vi "Gather image parameters.vi"(8 "error in":errorcluster, 11 "Acq params":T1) -> (0 "error out":errorcluster, 3 "Acqusition string":string)   [LabVIEW 2018]
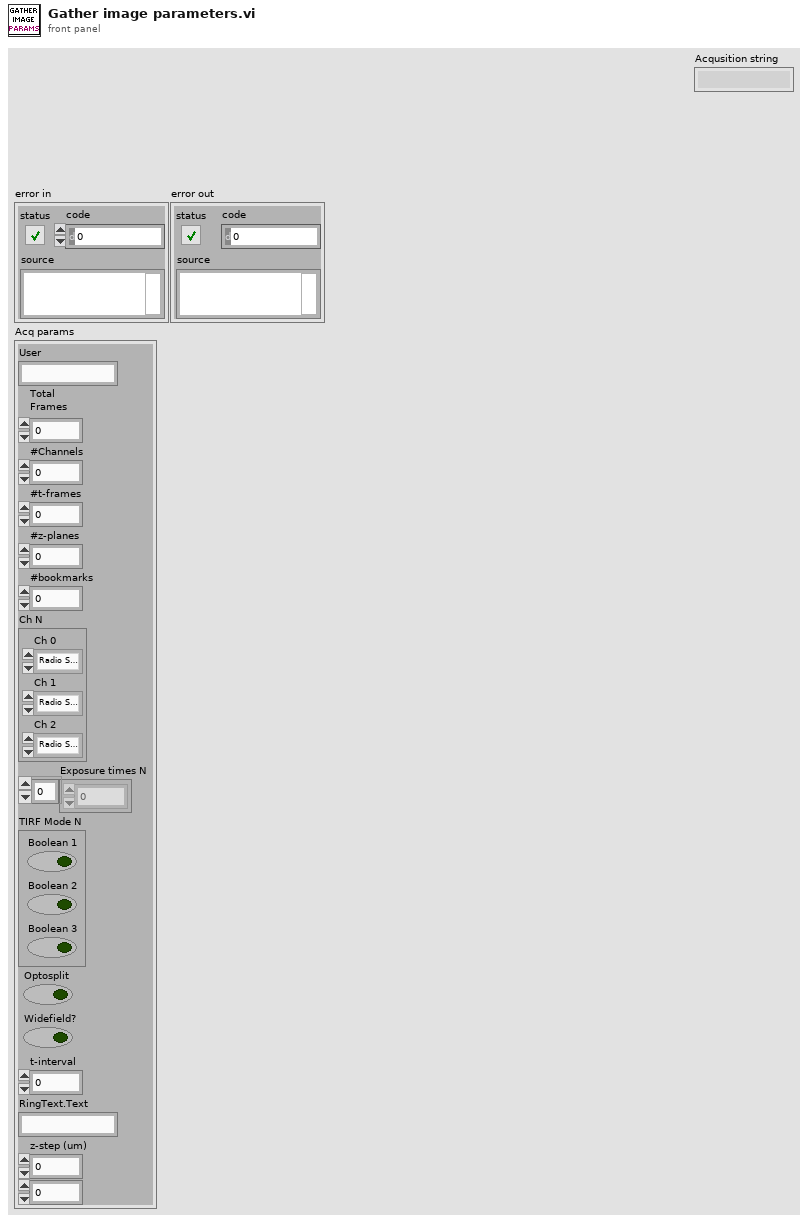
[diagram p1: front panel]
types:
  T1 = cluster{"User":string, "Total\nFrames":i16, "#Channels":i16, "#t-frames":i16, "#z-planes":i16, "#bookmarks":i16, "Ch N":cluster{"Ch 0":enum32{"Radio Selection 1", "Radio Selection 2", "Radio Selection 3"}, "Ch 1":enum32{"Radio Selection 1", "Radio Selection 2", "Radio Selection 3"}, "Ch 2":enum32{"Radio Selection 1", "Radio Selection 2", "Radio Selection 3"}}, "Exposure times N":dbl[], "TIRF Mode N":cluster{"Boolean 1":bool, "Boolean 2":bool, "Boolean 3":bool}, "Optosplit":bool, "Widefield?":bool, "t-interval":u32, "RingText.Text":string, "z-step (um)":dbl, i32}
  T2 = cluster{"Ch 0":enum32{"Radio Selection 1", "Radio Selection 2", "Radio Selection 3"}, "Ch 1":enum32{"Radio Selection 1", "Radio Selection 2", "Radio Selection 3"}, "Ch 2":enum32{"Radio Selection 1", "Radio Selection 2", "Radio Selection 3"}}
  T3 = cluster{"Boolean 1":bool, "Boolean 2":bool, "Boolean 3":bool}
  T4 = enum32{"Radio Selection 1", "Radio Selection 2", "Radio Selection 3"}
  T5 = enum32{"Radio Selection 1", "Radio Selection 2", "Radio Selection 3"}[]
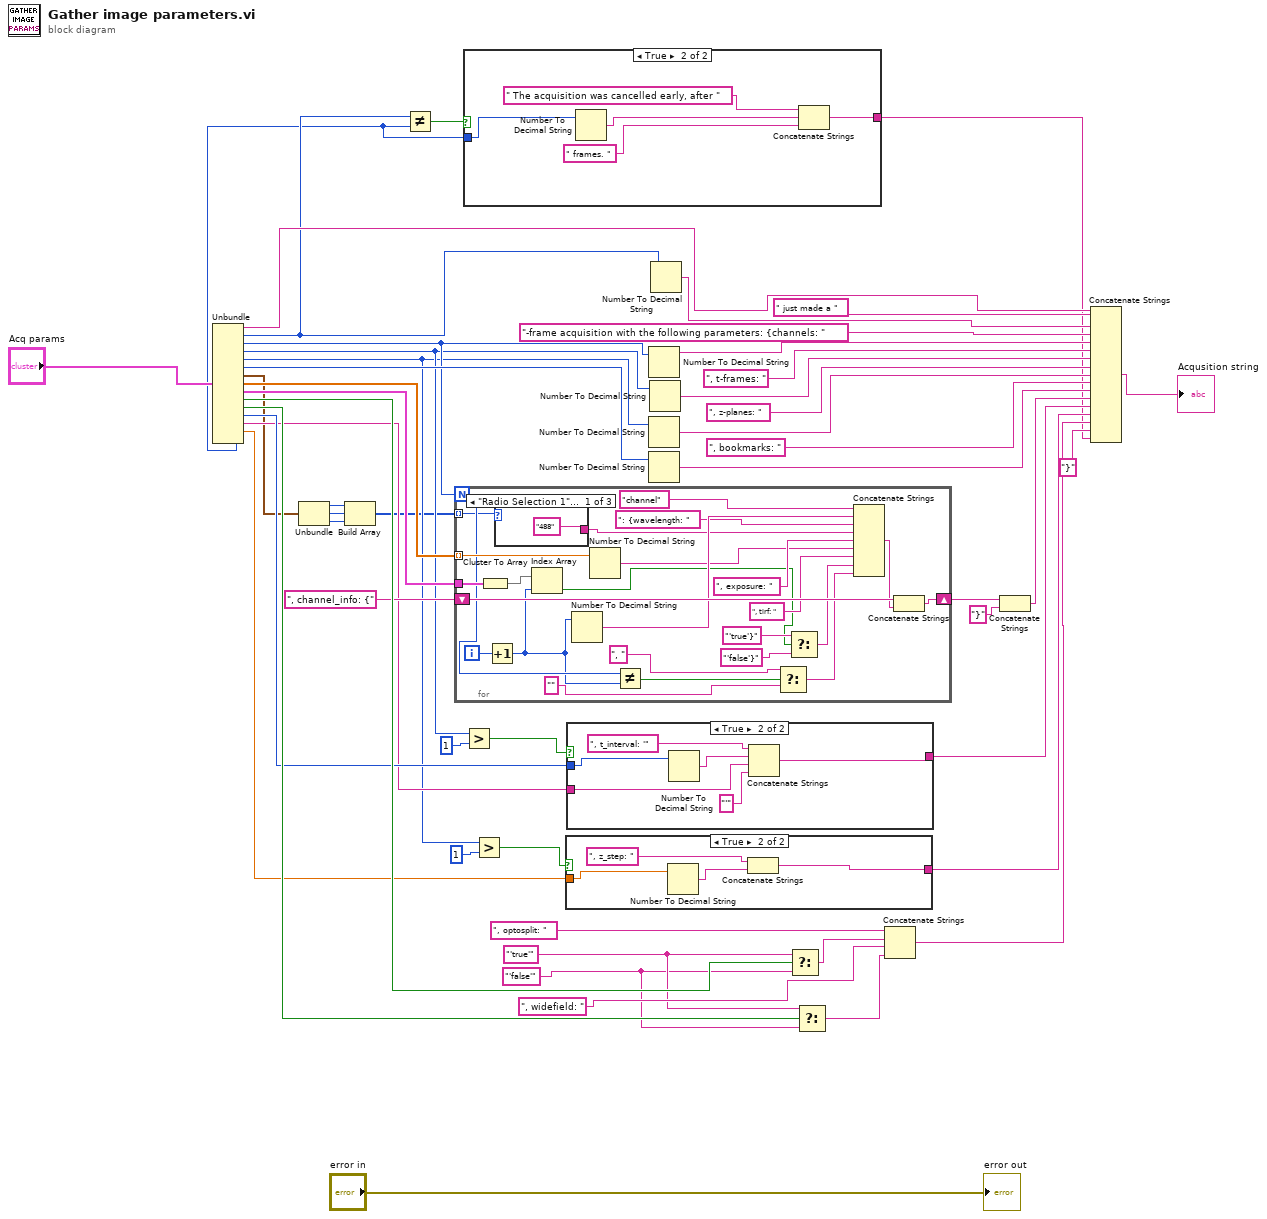
[diagram p0: block diagram]
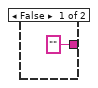
[diagram p2: hidden frame]
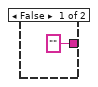
[diagram p3: hidden frame]
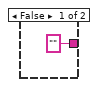
[diagram p4: hidden frame]
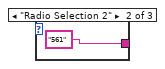
[diagram p5: hidden frame]
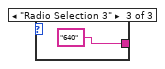
[diagram p6: hidden frame]
diagram:
  w16 = "'true'"
  w15 = "'false'"
  n1 = Unbundle("Acq params") -> ("User"=w42:string, "Total\nFrames"=w3:i16, "#Channels"=w37:i16, "#t-frames"=w33:i16, "#z-planes"=w21:i16, "#bookmarks"=w41:i16, "Ch N"=w11:T2, "Exposure times N"=w36:dbl[], "TIRF Mode N"=w35:T3, "Optosplit"=w38:bool, "Widefield?"=w39:bool, "t-interval"=w30:u32, "RingText.Text"=w29:string, "z-step (um)"=w24:dbl, w2:i32)
  n2 = Unbundle(w11) -> ("Ch 0"=w10:T4, "Ch 1"=w9:T4, "Ch 2"=w8:T4)
  n3 = Build Array(w10, w9, w8) -> (w7:T5)
  n4 = Not Equal?(x=w3, y=w2) -> (x != y?=w4:bool)
  n5 = for {
    N: w37 -> [w61]
    tunnel: w36 -> [w69] mode=indexing
    tunnel: w35 -> [w77]
    shift-right: [w75] -> w28
    shift-left: ", channel_info: {" -> [w74]
    tunnel: w7 -> [w54] mode=indexing
    i -> [w56]
    n6 = Cluster To Array(cluster=w77) -> (array=w76:bool[])
    n7 = Increment(x=w56) -> (x+1=w55:i32)
    n8 = case shown="\"Radio Selection 1\", Default" w54 {
      tunnel: ["488" ("string") "561" ("string") "640" ("string")] -> w53
      frame "Radio Selection 1", Default {
      }
      frame "Radio Selection 2" {
      }
      frame "Radio Selection 3" {
      }
    }
    n9 = Index Array(array=w76, index=w55) -> (element=w62:bool)
    n10 = Number To Decimal String(number=w55) -> (decimal integer string=w72:string)  [unwired: 1 in]
    n11 = Number To Decimal String(number=w69) -> (decimal integer string=w67:string)  [unwired: 1 in]
    n12 = Not Equal?(x=w61, y=w55) -> (x != y?=w60:bool)
    n13 = Select(t=", " ("string"), s=w60, f="" ("string")) -> (s? t:f=w59:string)
    n14 = Select(t="'true'}" ("string"), s=w62, f="'false'}" ("string")) -> (s? t:f=w65:string)
    n15 = Concatenate Strings("channel" ("string"), w72, ": {wavelength: " ("string"), w53, ", exposure: " ("string"), w67, ", tirf: " ("string"), w65, w59) -> (w70:string)
    n16 = Concatenate Strings(w74, w70) -> (w75:string)
  }
  n17 = case shown="True" w4 {
    tunnel: w2 -> [_ w86]
    tunnel: ["" w82] -> w1
    frame False {
    }
    frame True {
      n18 = Number To Decimal String(number=w86) -> (decimal integer string=w84:string)  [unwired: 1 in]
      n19 = Concatenate Strings(" The acquisition was cancelled early, after ", w84, " frames. ") -> (w82:string)
    }
  }
  n20 = Greater?(x=w33, y=i16 1) -> (0:w32:bool)
  n21 = Greater?(x=w21, y=i16 1) -> (0:w22:bool)
  n22 = case shown="True" w22 {
    tunnel: w24 -> [_ w90]
    tunnel: ["" w88] -> w20
    frame False {
    }
    frame True {
      n23 = Number To Decimal String(number=w90) -> (decimal integer string=w89:string)  [unwired: 1 in]
      n24 = Concatenate Strings(", z_step: ", w89) -> (w88:string)
    }
  }
  n25 = case shown="True" w32 {
    tunnel: w30 -> [_ w97]
    tunnel: w29 -> [_ w95]
    tunnel: ["" w93] -> w25
    frame False {
    }
    frame True {
      n26 = Number To Decimal String(number=w97) -> (decimal integer string=w96:string)  [unwired: 1 in]
      n27 = Concatenate Strings(", t_interval: '", w96, w95, "'" ("string")) -> (w93:string)
    }
  }
  n28 = Number To Decimal String(number=w37) -> (decimal integer string=w46:string)  [unwired: 1 in]
  n29 = Number To Decimal String(number=w21) -> (decimal integer string=w50:string)  [unwired: 1 in]
  n30 = Number To Decimal String(number=w41) -> (decimal integer string=w52:string)  [unwired: 1 in]
  n31 = Number To Decimal String(number=w33) -> (decimal integer string=w48:string)  [unwired: 1 in]
  n32 = Number To Decimal String(number=w3) -> (decimal integer string=w44:string)  [unwired: 1 in]
  n33 = Select(t=w16, s=w38, f=w15) -> (s? t:f=w18:string)
  n34 = Select(t=w16, s=w39, f=w15) -> (s? t:f=w14:string)
  n35 = Concatenate Strings(", optosplit: ", w18, ", widefield: ", w14) -> (w13:string)
  n36 = Concatenate Strings(w28, "}" ("string")) -> (w27:string)
  n37 = Concatenate Strings(w42, " just made a " ("string"), w44, "-frame acquisition with the following parameters: {channels: ", w46, ", t-frames: ", w48, ", z-planes: ", w50, ", bookmarks: ", w52, w27, w25, w20, w13, "}" ("string"), w1) -> (→"Acqusition string":string)
  "error out" <- "error in"
